vi "NI VeriStand - Add Custom Device Channel.vi"(4 "Property Values":variant[](array[variant]), 5 "Highlight? (F)":bool, 6 "Property names":string[](array[string]), 7 "GUID (Default Channel)":string="03D3BB99-1485-13A6-561D1F898F032919", 8 "error in (no error)":errorcluster, 9 "Channel":T2, 10 "Channel Name":string, 11 "Parent Ref in":T1 format="%.0x") -> (0 "error out":errorcluster, 1 "Channel Ref":T1 format="%.0x", 2 "Newly Created?":bool, 3 "Parent Ref out":T1 format="%.0x")   [LabVIEW 2020, in "Custom Device API.lvlib"]
doc: "Adds a channel to the device or device subsection specified by <B>Parent Ref in</B>. If the <B>Channel Name</B> you specify already exists, this VI updates the <B>Channel</B> information (<B>Type</B>, <B>Units</B>, etc.), properties, and the <B>GUID</B> for the configuration page."
uses:
  <vilib>/NI VeriStand/Custom Device API/Custom Device API.lvlib
  <vilib>/NI VeriStand/Custom Device API/Custom Device Item Ref.ctl
  <vilib>/NI VeriStand/Custom Device API/Custom Device Channel.ctl
  <vilib>/NI VeriStand/Custom Device API/Custom Device Channel Type.ctl
  4607a54e-09dc-41a6-b753-4646183d2ed6.vi
  <vilib>/NI VeriStand/Custom Device API/Custom Device Offline Path.vi
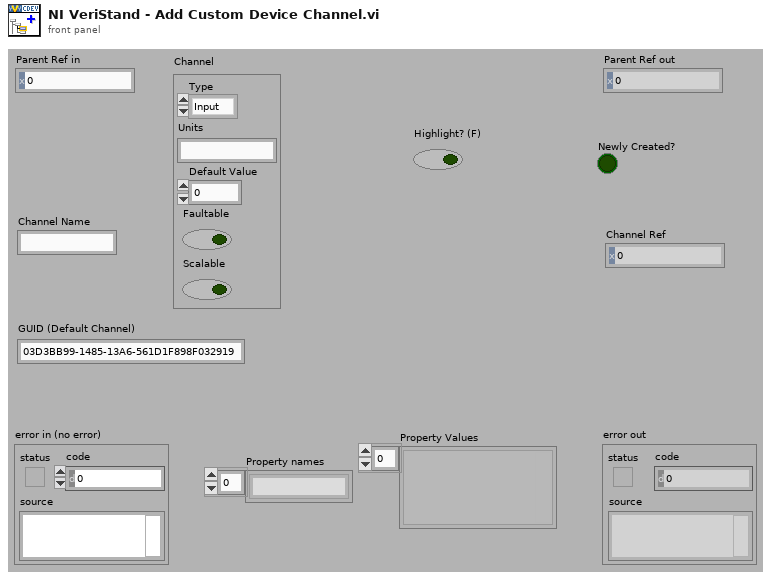
[diagram p1: front panel]
types:
  T1 = typedef "Custom Device API.lvlib/Custom Device Item Ref.ctl" = u64
  T2 = typedef "Custom Device API.lvlib/Custom Device Channel.ctl" = cluster{"Type":T3, "Units":string, "Default Value":dbl, "Faultable":bool, "Scalable":bool}
  T3 = typedef "Custom Device API.lvlib/Custom Device Channel Type.ctl" = enum16{"Input", "Output"}
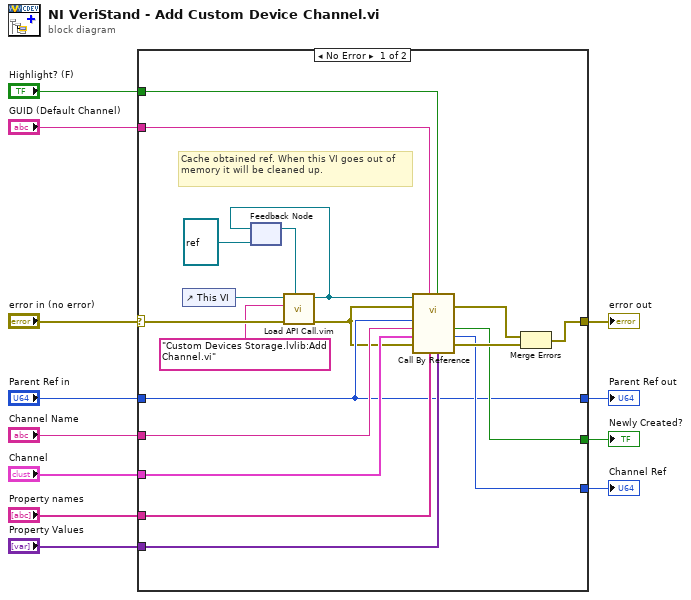
[diagram p0: block diagram]
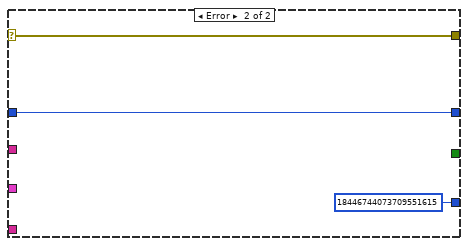
[diagram p2: hidden frame]
diagram:
  n1 = case shown="No Error" "error in (no error)" {
    selector: "error in (no error)" -> [w17 w34]
    tunnel: "GUID (Default Channel)" -> [w30 _]
    tunnel: "Highlight? (F)" -> [w29 _]
    tunnel: [w28 T1 18446744073709551615 ("Channel Ref")] -> w10
    tunnel: [w27 w34] -> w9
    tunnel: [w20 w32] -> w8
    tunnel: "Property Values" -> [w26 _]
    tunnel: "Property names" -> [w25 _]
    tunnel: "Parent Ref in" -> [w20 w32]
    tunnel: "Channel Name" -> [w24 _]
    tunnel: "Channel" -> [w23 _]
    tunnel: [w22 _] -> w2
    frame No Error {
      # "Cache obtained ref. When this VI goes out of memory it will be cleaned up."
      n2 = control-ref of="This VI"() -> (w18:refnum<vi>)
      n3 = feedback #1(refnum<vi> refnum ("type specifier VI Refnum (for type only)")) -> (w19:refnum<vi>)
      n4 = call "Load API Call.vim"("VI reference in"=w19, "error in (no error)"=w17, "VI qualified name"="Custom Devices Storage.lvlib:Add Channel.vi", "Caller VI ref"=w18) -> ("error out"=w16:errorcluster, "VI reference"=w15:refnum<vi>)  [unwired: 6 in]
      n5 = feedback-in #1(w15) -> ()
      n6 = call-by-ref "?"(reference=w15, error in=w16, "Property Values"=w26, "Highlight? (F)"=w29, "Property names"=w25, "GUID (Default Channel)"=w30, 8:"error in (no error)"=w16, "Channel"=w23, "Channel Name"=w24, "Parent Ref in"=w20) -> (error out=w21:errorcluster, 0:"error out"=w31:errorcluster, "Channel Ref"=w28:T1, "Newly Created?"=w22:bool)  [unwired: 2 out]
      n7 = Merge Errors(w21, w31) -> (w27:errorcluster)
    }
    frame Error {
    }
  }
  "Parent Ref out" <- w8
  "error out" <- w9
  "Channel Ref" <- w10
  "Newly Created?" <- w2
